vi "State2_old.vi"(0 "Start":bool, 1 "Stop":bool, 2 "Reset":bool, 3 "C":bool[][](array[boolean]), 4 "Stage table":u32[][](array[numeric])=[[3000, 1, 2, 2], [3000, 2, 3, 3], [3000, 3, 4, 4], [3000, 0, 0, 0]], 7 "End step":u32=4, 9 "Descriptions":string[](array[string])) -> (13 "Description":string, 14 "Start":bool, 15 "Stop":bool, 16 "End":bool, 17 "t":u32, 18 "N curr":u32)   [LabVIEW 2015]
uses:
  Userlib.lvlib
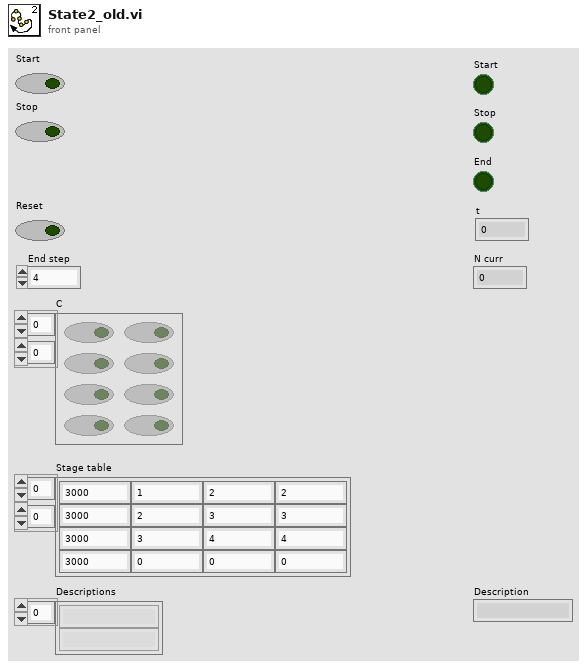
[diagram p1: front panel]
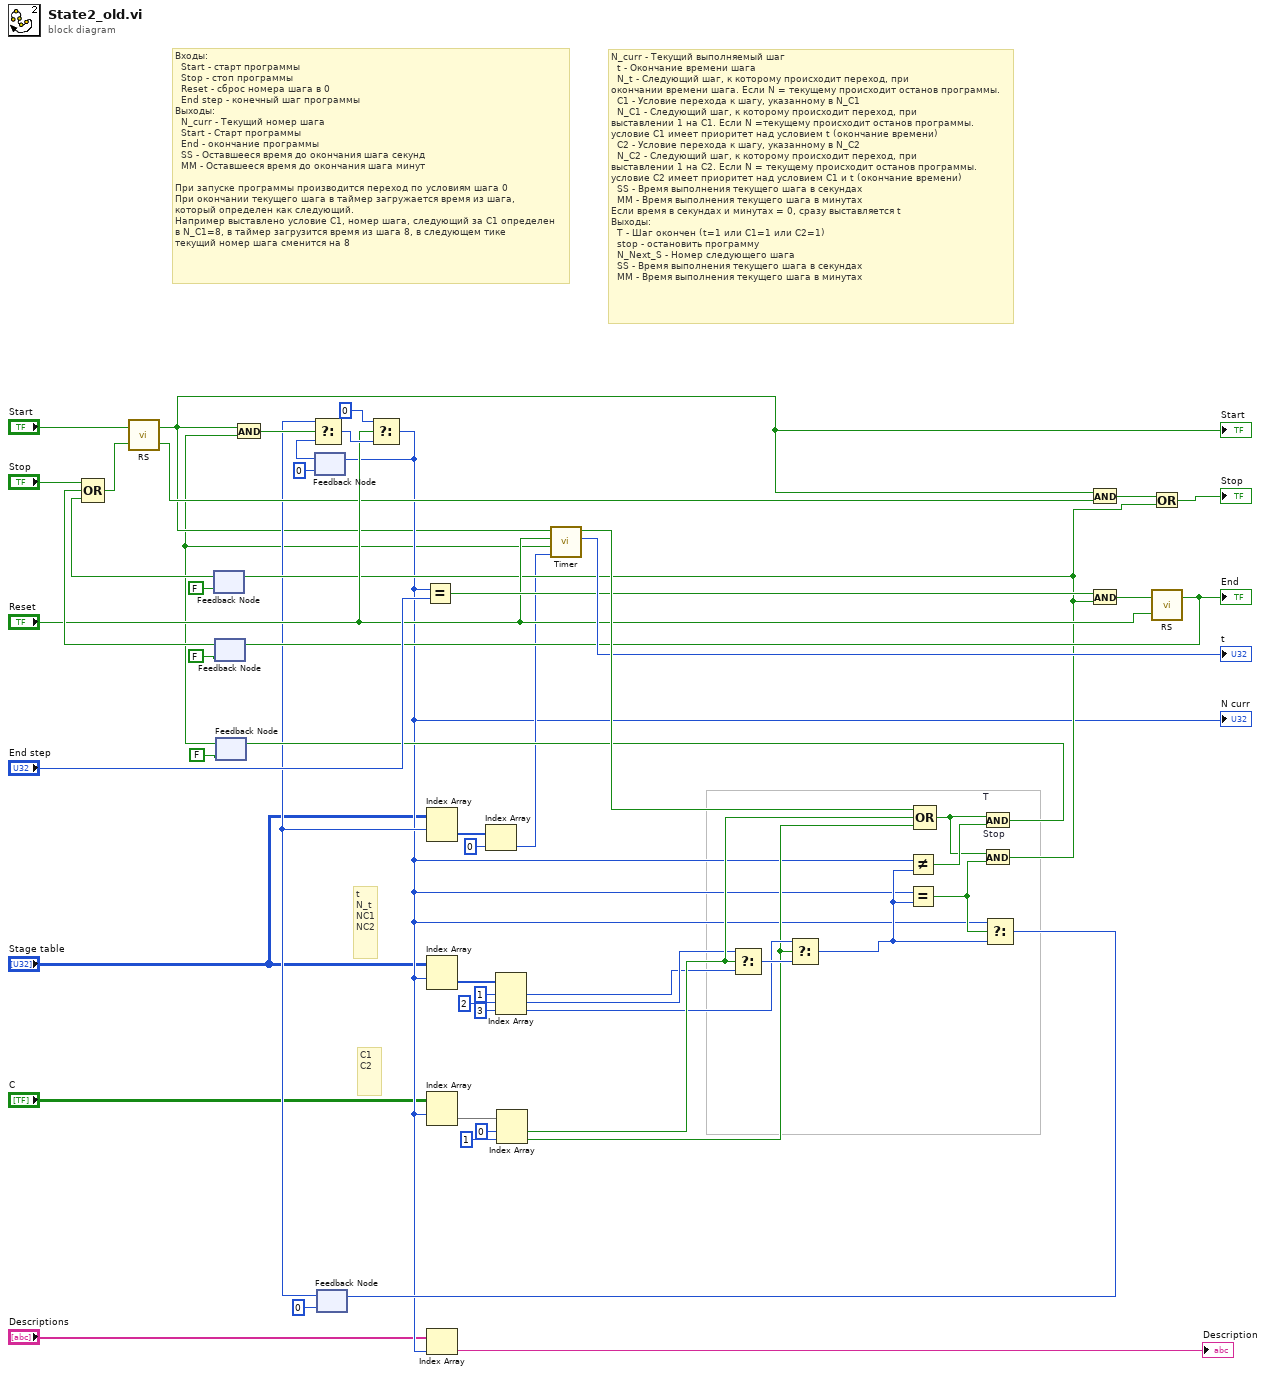
[diagram p0: block diagram]
diagram:
  # "C1\nC2"
  # "t\nN_t\nNC1\nNC2"
  # "N_curr - Текущий выполняемый шаг\n  t - Окончание времени шага\n  N_t - Следующий шаг, к которому происходит переход, при\nокончании времени шага. Если N = текущему происходит останов программы.\n  C1 - Условие перехода к шагу, указанному в N_C1\n  N_C1 - Следующий шаг, к которому происходит переход, при\nвыставлении 1 на С1. Если N =текущему происходит останов программы.\nусловие С1 имеет приоритет над условием t (окончание времени)\n  C2 - Условие перехода к шагу, указанному в N_C2\n  N_C2 - Следующий шаг, к которому происходит переход, при\nвыставлении 1 на С2. Если N = текущему происходит останов программы.\nусловие С2 имеет приоритет над условием С1 и t (окончание времени)\n  SS - Время выполнения текущего шага в секундах\n  MM - Время выполнения текущего шага в минутах\nЕсли время в секундах и минутах = 0, сразу выставляется t\nВыходы:\n  T - Шаг окончен (t=1 или C1=1 или С2=1)\n  stop - остановить программу\n  N_Next_S - Номер следующего шага\n  SS - Время выполнения текущего шага в секундах\n  MM - Время выполнения текущего шага в минутах"
  # "Входы:\n  Start - старт программы\n  Stop - стоп программы\n  Reset - сброс номера шага в 0\n  End step - конечный шаг программы\nВыходы:\n  N_curr - Текущий номер шага\n  Start - Старт программы\n  End - окончание программы\n  SS - Оставшееся время до окончания шага секунд\n  MM - Оставшееся время до окончания шага минут\n\nПри запуске программы производится переход по условиям шага 0\nПри окончании текущего шага в таймер загружается время из шага,\nкоторый определен как следующий.\nНапример выставлено условие C1, номер шага, следующий за С1 определен\nв N_C1=8, в таймер загрузится время из шага 8, в следующем тике \nтекущий номер шага сменится на 8"
  n1 = feedback #1(FALSE ("Q")) -> (w40:bool)
  n2 = feedback #2(FALSE ("Q")) -> (w39:bool)
  n3 = Compound Arithmetic op=OR("Stop", w39, w40) -> (w54:bool)
  n4 = call "RS.vi"("R"=w54, "S"="Start") -> ("~Q"=w26:bool, "Q"=w2:bool)
  "Start" <- w2
  n5 = feedback #3(FALSE ("Q")) -> (w1:bool)
  n6 = And(x=w2, y=w1) -> (x .and. y?=w55:bool)
  n7 = feedback #4(u32 0) -> (w33:u32)
  n8 = feedback #5(u32 0) -> (w24:u32)
  n9 = Select(t=w24, s=w55, f=w33) -> (s? t:f=w35:u32)
  n10 = Select(t=u32 0, s="Reset", f=w35) -> (s? t:f=w6:u32)
  "N curr" <- w6
  n11 = feedback-in #4(w6) -> ()
  n12 = Equal?(x=w6, y="End step") -> (x = y?=w29:bool)
  n13 = Index Array(array="Stage table", index (row)=w24) -> (element=w23:u32[])  [unwired: 1 in]
  n14 = Index Array(array="Stage table", index (row)=w6) -> (element=w19:u32[])  [unwired: 1 in]
  n15 = Index Array(array="C", index (row)=w6) -> (element=w18:bool[])  [unwired: 1 in]
  n16 = Index Array(array="Descriptions", index=w6) -> (element=→"Description":string)
  n17 = Index Array(array=w23, index=0) -> (element=w22:u32)
  n18 = Index Array(array=w19, index #1=1 ("index"), index #2=2 ("index"), index #3=3 ("index")) -> (element #1=w9:u32, element #2=w10:u32, element #3=w13:u32)
  n19 = Index Array(array=w18, index #1=0 ("index"), index #2=1 ("index")) -> (element #1=w16:bool, element #2=w7:bool)
  n20 = call "Timer.vi"("ms"=w22, "Load"=w1, "Reset"="Reset", "Start"=w2) -> ("t ms"=→"t":u32, "End"=w44:bool)  [unwired: 5 in]
  n21 = Select(t=w10, s=w16, f=w9) -> (s? t:f=w48:u32)
  n22 = Select(t=w13, s=w7, f=w48) -> (s? t:f=w15:u32)
  n23 = Not Equal?(x=w6, y=w15) -> (x != y?=w47:bool)
  n24 = Equal?(x=w6, y=w15) -> (x = y?=w45:bool)
  n25 = Compound Arithmetic op=OR(w44, w16, w7) -> (w46:bool)
  n26 = And "T"(x=w46, y=w47) -> (x .and. y?=w42:bool)
  n27 = feedback-in #3(w42) -> ()
  n28 = And "Stop"(x=w46, y=w45) -> (x .and. y?=w25:bool)
  n29 = feedback-in #1(w25) -> ()
  n30 = Select(t=w6, s=w45, f=w15) -> (s? t:f=w36:u32)
  n31 = feedback-in #5(w36) -> ()
  n32 = And(x=w2, y=w26) -> (x .and. y?=w28:bool)
  n33 = And(x=w29, y=w25) -> (x .and. y?=w51:bool)
  n34 = Or(x=w28, y=w25) -> (x .or. y?=→"Stop":bool)
  n35 = call "RS.vi"("R"="Reset", "S"=w51) -> ("Q"=w30:bool)  [unwired: 1 out]
  "End" <- w30
  n36 = feedback-in #2(w30) -> ()
